vi "Discard Packet.vi"(8 "error in (no error)":errorcluster, 10 "Ack":refnum<class "Ack.lvclass">, 11 "Subscription in":refnum<class "Subscription.lvclass">) -> (0 "error out":errorcluster, 1 "Discarded":bool, 2 "Ack dup":refnum<class "Ack.lvclass">, 3 "Subscription out":refnum<class "Subscription.lvclass">)   [LabVIEW 2013, in "MQTT Server.lvlib" / "Subscription.lvclass"]
uses:
  Subscription.lvclass
  <vilib>/LabVIEW Open Source Project/MQTT Control Packets/Control Packets/Ack/Ack.lvclass
  Subscription.lvclass/Subscription.ctl
  <vilib>/LabVIEW Open Source Project/MQTT Control Packets/Control Packets/ControlPacket/ControlPacket.lvclass/ControlPacket.ctl
  <vilib>/LabVIEW Open Source Project/MQTT Control Packets/Control Packets/ControlPacket/ControlPacket.lvclass
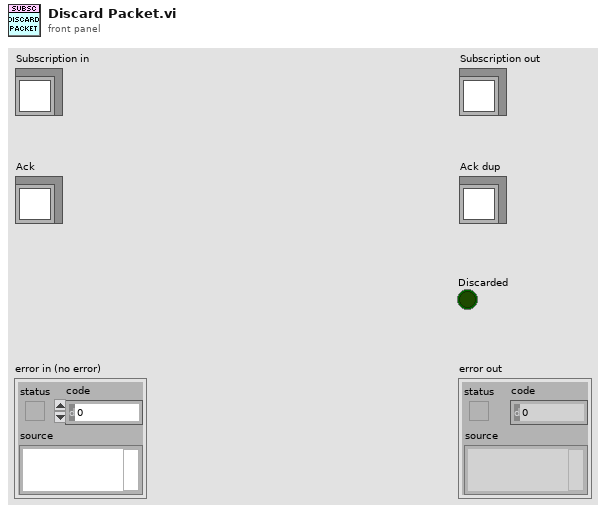
[diagram p1: front panel]
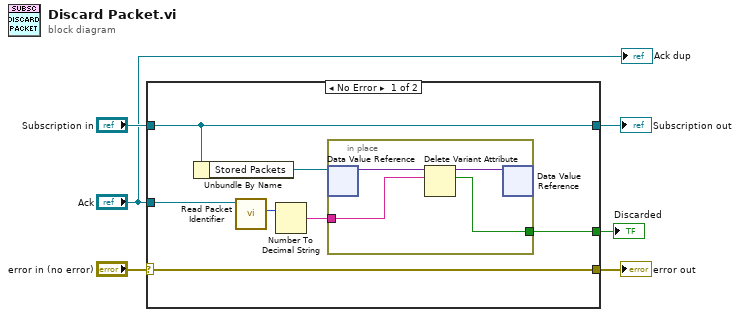
[diagram p0: block diagram]
diagram:
  n1 = case shown="No Error" "error in (no error)" {
    selector: "error in (no error)" -> [w13 w19]
    tunnel: [w13 w19] -> w5
    tunnel: [w12 w18] -> w3
    tunnel: "Subscription in" -> [w12 w18]
    tunnel: "Ack" -> [w10 _]
    tunnel: [w7 _] -> w2
    frame No Error {
      n2 = Unbundle By Name(w12) -> ("Stored Packets"=w11:refnum<data-value>)
      n3 = call <vilib>:"Read Packet Identifier.vi"("ControlPacket in"=w10) -> ("Packet Identifier"=w9:u16)  [unwired: 9 in, 1 out]
      n4 = Number To Decimal String(number=w9) -> (decimal integer string=w8:string)  [unwired: 1 in]
      n5 = in-place {
        in-place-border: w8 -> [w15]
        in-place-border: [w14] -> w7
        n6 = in-place-dvr #1(w11) -> (w17:variant)  [unwired: 1 out]
        n7 = Delete Variant Attribute(6:w15, 7:w17) -> (2:w14:bool, 3:w16:variant)  [unwired: 1 in, 1 out]
        n8 = in-place-dvr #1(w16) -> ()  [unwired: 2 out]
      }
    }
    frame Error {
    }
  }
  "error out" <- w5
  "Subscription out" <- w3
  "Discarded" <- w2
  "Ack dup" <- "Ack"
